vi "AVI-Viewer UI initialisation.vi"(6 "I16 image ref in":T4, 7 "AVI modes refs in":T1, 8 "error in (no error)":errorcluster, 9 "RGB image ref in":T4, 10 "AVI File Path":path, 11 "Queue in":refnum<queue>) -> (0 "error out":errorcluster, 1 "AVI modes refs out":T1, 2 "Number of Frames":u32, 3 "Refnum out":T4, 5 "Scrollbar position":i32)   [LabVIEW 2020]
uses:
  Typedefs/Speed Viewer States enum.ctl
  <vilib>/vision/Image Controls.llb/IMAQ Image.ctl
  Typedefs/AVI modes refs cluster.ctl
  <vilib>/vision/Avi1.llb/AviRefnum.ctl
  <vilib>/vision/Avi.llb/IMAQ AVI2 Refnum.ctl
  Globals/gl_Time series viewer globals.vi
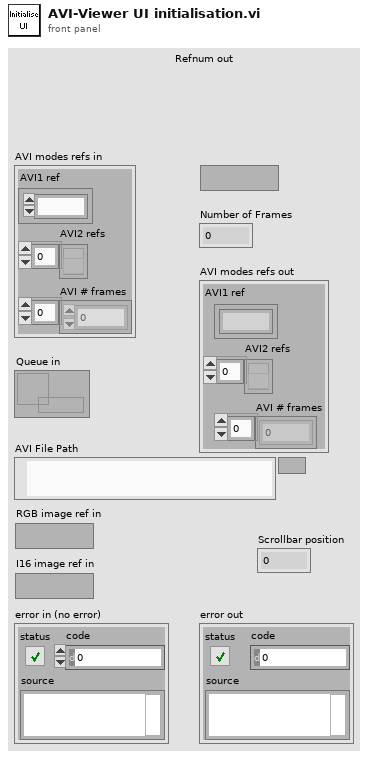
[diagram p1: front panel]
types:
  T1 = typedef "AVI modes refs cluster.ctl" = cluster{"AVI1 ref":T2, "AVI2 refs":T3[], "AVI # frames":u32[]}
  T2 = typedef "AviRefnum.ctl" = refnum<k1>
  T3 = typedef "IMAQ AVI2 Refnum.ctl" = refnum<k20>
  T4 = typedef "IMAQ Image.ctl" = refnum<image>
  T5 = enum8{"Enabled", "Disabled", "Disabled and Grayed Out"}
  T6 = typedef "Time series viewer refs.ctl" = cluster{"This VI":refnum<vi>, "Image control":refnum<vi>, "AVI Mode ind":refnum<vi>, "Play":refnum<vi>, "Stop":refnum<vi>, "Back":refnum<vi>, "Scrollbar":refnum<vi>, "Video length info":refnum<vi>, "Expected speed values":refnum<vi>, "Intensity":refnum<vi>, "Path":refnum<vi>, "Selection sliders":refnum<vi>, "Speed Graph ref":refnum<vi>, "Frame rate set (fps)":refnum<vi>, "Number of rows to generate":refnum<vi>, "VL Image Array":refnum<vi>, "Image Scrollbar":refnum<vi>, "Channel to load":refnum<vi>, "Colour":refnum<vi>}
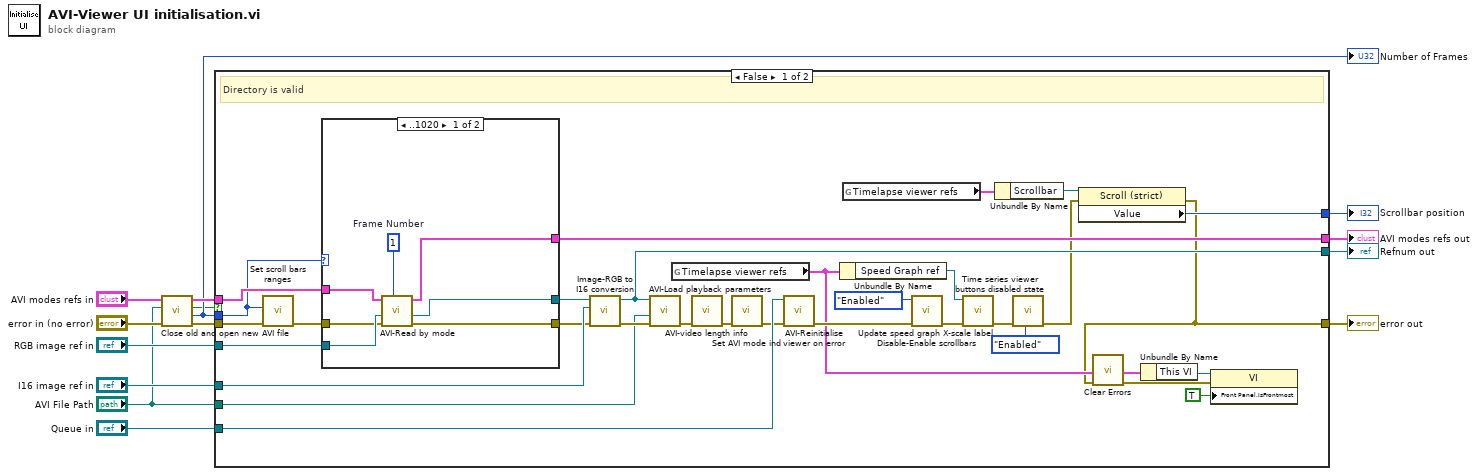
[diagram p0: block diagram]
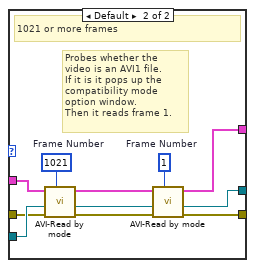
[diagram p2: hidden frame]
diagram:
  n1 = call "Close old and open new AVI file.vi"("error in (no error)"="error in (no error)", "AVI File Path"="AVI File Path", "AVI modes refs"="AVI modes refs in") -> ("error out"=w11:errorcluster, "Number of Frames"=w4:u32, "Cancelled due to the selected \nAVI file being located within an\n\"Exported 8-bit videos\" directory!"=w2:bool, "AVI modes refs"=w8:T1)  [unwired: 4 in, 1 out]
  "Number of Frames" <- w4
  n2 = case shown="False" w2 {
    tunnel: "Queue in" -> [w42 _]
    tunnel: "RGB image ref in" -> [w40 _]
    tunnel: w11 -> [w39 w64]
    tunnel: "I16 image ref in" -> [w38 _]
    tunnel: [w34 w65] -> w9
    tunnel: w8 -> [w33 w65]
    tunnel: "AVI File Path" -> [w32 _]
    tunnel: [w31 _] -> w5
    tunnel: w4 -> [w29 _]
    tunnel: [w15 w64] -> w3
    tunnel: [w17 _] -> w1
    frame False {
      # "Directory is valid"
      n3 = call "Set scroll bars ranges.vi"("error in (no error)"=w39, "Number of frames"=w29) -> ("error out"=w37:errorcluster)  [unwired: 9 in]
      n4 = case shown="..1020" w29 {
        tunnel: w40 -> [w52 w63]
        tunnel: w37 -> [w51 w62]
        tunnel: [w49 w59] -> w36
        tunnel: [w48 w57] -> w35
        tunnel: [w47 w55] -> w34
        tunnel: w33 -> [w46 w60]
        frame ..1020 {
          w50 = 1  # Frame Number
          n5 = call "AVI-Read by mode.vi"("Frame number (unity-based)"=w50, "error in (no error)"=w51, "RGB image ref in"=w52, "AVI modes refs"=w46) -> ("error out"=w49:errorcluster, "RGB image ref out"=w48:T4, "AVI modes refs"=w47:T1)  [unwired: 5 in]
        }
        frame Default {
          w54 = 1  # Frame Number
          w61 = 1021  # Frame Number
          # "Probes whether the video is an AVI1 file.\nIf it is it pops up the compatibility mode option window.\nThen it reads frame 1."
          # "1021 or more frames"
          n6 = call "AVI-Read by mode.vi"("Frame number (unity-based)"=w61, "error in (no error)"=w62, "RGB image ref in"=w63, "AVI modes refs"=w60) -> ("error out"=w53:errorcluster, "RGB image ref out"=w58:T4, "AVI modes refs"=w56:T1)  [unwired: 5 in]
          n7 = call "AVI-Read by mode.vi"("Frame number (unity-based)"=w54, "error in (no error)"=w53, "RGB image ref in"=w58, "AVI modes refs"=w56) -> ("error out"=w59:errorcluster, "RGB image ref out"=w57:T4, "AVI modes refs"=w55:T1)  [unwired: 5 in]
        }
      }
      n8 = call "Image-RGB to I16 conversion.vi"("error in (no error)"=w36, "I16 image ref in"=w38, "RGB image ref in"=w35) -> ("error out"=w44:errorcluster, "I16 image ref out"=w31:T4)  [unwired: 7 in]
      n9 = call "AVI-Load playback parameters.vi"("error in (no error)"=w44, "AVI File Path"=w32, "I16 image ref"=w31) -> ("error out"=w43:errorcluster)  [unwired: 8 in]
      n10 = global read "gl_Time series viewer globals.vi" "Timelapse viewer refs"() -> (w21:T6)
      n11 = call "AVI-video length info.vi"("error in (no error)"=w43) -> ("error out"=w45:errorcluster)  [unwired: 8 in, 2 out]
      n12 = call "Set AVI mode ind.vi"("error in (no error)"=w45) -> ("error out"=w41:errorcluster)  [unwired: 10 in]
      n13 = call "AVI-Reinitialise viewer on error.vi"("error in (no error)"=w41, "Queue in"=w42) -> ("error out"=w30:errorcluster)  [unwired: 9 in]
      n14 = Unbundle By Name(w21) -> ("Speed Graph ref"=w27:refnum<vi>)
      n15 = global read "gl_Time series viewer globals.vi" "Timelapse viewer refs"() -> (w19:T6)
      n16 = call "Disable-Enable scrollbars.vi"("error in (no error)"=w30, "Disabled state"=T5."Enabled") -> ("error out"=w28:errorcluster)  [unwired: 9 in]
      n17 = call "Update speed graph X-scale label.vi"("error in (no error)"=w28, "Speed Graph"=w27) -> ("error out"=w22:errorcluster)  [unwired: 9 in]
      n18 = Unbundle By Name(w19) -> ("Scrollbar"=w18:refnum<vi>)
      n19 = call "Time series viewer buttons disabled state.vi"("error in (no error)"=w22, "Disabled"=T5."Enabled") -> ("error out"=w16:errorcluster)  [unwired: 9 in]
      n20 = property class="Scroll (strict)"(reference=w18, error in=w16) -> (error out=w15:errorcluster, "Value"=w17:i32)  [unwired: 1 out]
      n21 = call <vilib>:"Clear Errors.vi"("error in (no error)"=w15) -> ("error out"=w24:errorcluster)  [unwired: 5 in, 1 out]
      n22 = Unbundle By Name(w21) -> ("This VI"=w20:refnum<vi>)
      n23 = property on="Property Node" class="VI"(reference=w20, error in=w24, "Front Panel.IsFrontmost"=TRUE ("Front Panel Window:Is Frontmost")) -> ()  [unwired: 2 out]
    }
    frame True {
      # "Cancelled due to the selected AVI file being located within an \"Exported 8-bit videos\" directory!"
    }
  }
  "error out" <- w3
  "Refnum out" <- w5
  "AVI modes refs out" <- w9
  "Scrollbar position" <- w1
